vi "Tstabilizzazione auto.vi"() -> ()   [LabVIEW 2019]
panel:
  in  "Tempo stabilizzazione [s]":dbl
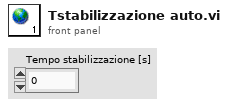
[diagram p1: front panel]
diagram:
